vi "DistanceFromCenter.vi"(9 "y":dbl, 10 "x":dbl) -> (2 "distance":dbl)   [LabVIEW 2012]
uses:
  <vilib>/imath/engines/lvmath2/RunTimeEngine/NodeEndStatement/NIMS_NodeEndStatement_Output.vi
  <instcachedir>/0/NIMS_NodeEndStatement_Output_53EC0D466D134D7ABD903AC30B43404B.lvgen/NIMS_NodeEndStatement_Output_53EC0D466D134D7ABD903AC30B43404B_010.vi
  <vilib>/imath/engines/lvmath2/RunTimeEngine/ErrorHandling/NIMS_Finalize Error.vi
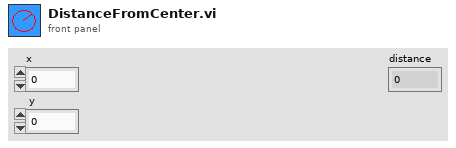
[diagram p1: front panel]
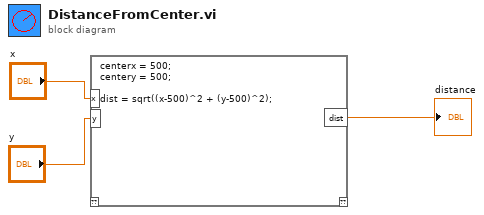
[diagram p0: block diagram]
diagram:
  n1 = mathscript code="centerx = 500;\ncentery = 500;\n\ndist = sqrt((x-500)^2 + (y-500)^2);"("x"="x", "y"="y") -> ("dist"=→"distance":cdb)  [unwired: 1 in, 1 out]
